vi "Initialize Counter Task.vi"(8 "error in (no error)":errorcluster, 11 "BNT_ULx-MCSV in":refnum<class "BNT_ULx-MCSV.lvclass">) -> (0 "error out":errorcluster, 3 "Counter ULx Task":refnum<k24>)   [LabVIEW 2021, in "BNT_ULx.lvlib" / "BNT_ULx-MCSV.lvclass"]
doc: "Initialize ULx Counter task.\n\n<b>Default Implementation:</b> Count Edges\n\nThis dynamic dispatch VI can be overritten by derived classes to implement other counter tasks."
uses:
  BNT_ULx-MCSV.lvclass
  <vilib>/ULx/ULx_LV.dll
  BNT_ULx-MCSV.lvclass/BNT_ULx-MCSV.ctl
  <vilib>/ULx/Create Channel.llb/ULx Create Channel (CI-Count Edges).vi
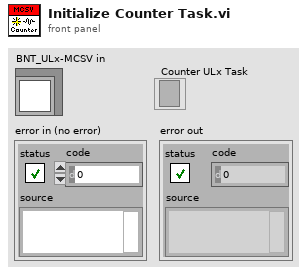
[diagram p1: front panel]
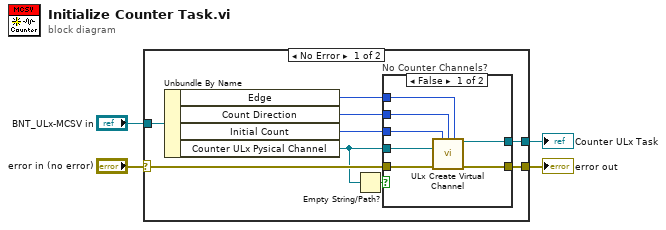
[diagram p0: block diagram]
diagram:
  n1 = case shown="No Error" "error in (no error)" {
    selector: "error in (no error)" -> [w7 w22]
    tunnel: [w12 w22] -> w3
    tunnel: "BNT_ULx-MCSV in" -> [w8 _]
    tunnel: [w11 _] -> w1
    frame No Error {
      n2 = Unbundle By Name(w8) -> ("Edge"=w13:i32, "Count Direction"=w10:i32, "Initial Count"=w9:u32, "Counter ULx Pysical Channel"=w5:refnum<k21>)
      n3 = Empty String/Path?(string/path=w5) -> (empty?=w6:bool)
      n4 = case "No Counter Channels?" shown="False" w6 {
        tunnel: w13 -> [w15 _]
        tunnel: w5 -> [w18 _]
        tunnel: [w19 w21] -> w12
        tunnel: [w17 _] -> w11
        tunnel: w10 -> [w14 _]
        tunnel: w9 -> [w16 _]
        tunnel: w7 -> [w20 w21]
        frame False {
          n5 = call-poly <vilib>:"ULx Create Virtual Channel.vi"("initial count"=w16, "count direction"=w14, "edge"=w15, "counters"=w18, "error in"=w20) -> ("task out"=w17:refnum<k24>, "error out"=w19:errorcluster)  [unwired: 9 in]
        }
        frame True {
        }
      }
    }
    frame Error {
    }
  }
  "error out" <- w3
  "Counter ULx Task" <- w1
